vi "Launcher Template (Top Level VI).vi"() -> ()   [LabVIEW 2021]
uses:
  Typedefs/FGV Ref. Modules Function.ctl
  Typedefs/Enum_Module_Name.ctl
  Typedefs/Module References.ctl
  Typedefs/Message.ctl
  Modules/Configuration/Main Config.vi
  Modules/Core UI/SubVIs/Main Core UI.vi
  Modules/Module Template/SubVIs/Main.vi
  Modules/Module Template/Module Template.lvlib
  Modules/Configuration/Configuration.lvlib
  Architecture.lvlib
  Modules/Core UI/Core UI.lvlib
panel:
  out "error out":errorcluster
  in  "Loading Bar":u8(slide) caption="Loading Database..." max=100 step=1 scale=0.0..100.0
  # "APPLICATION LAUNCHER"
  # "Juan Pérez Rodríguez"
  # "https://CtrlVIStudios.com"
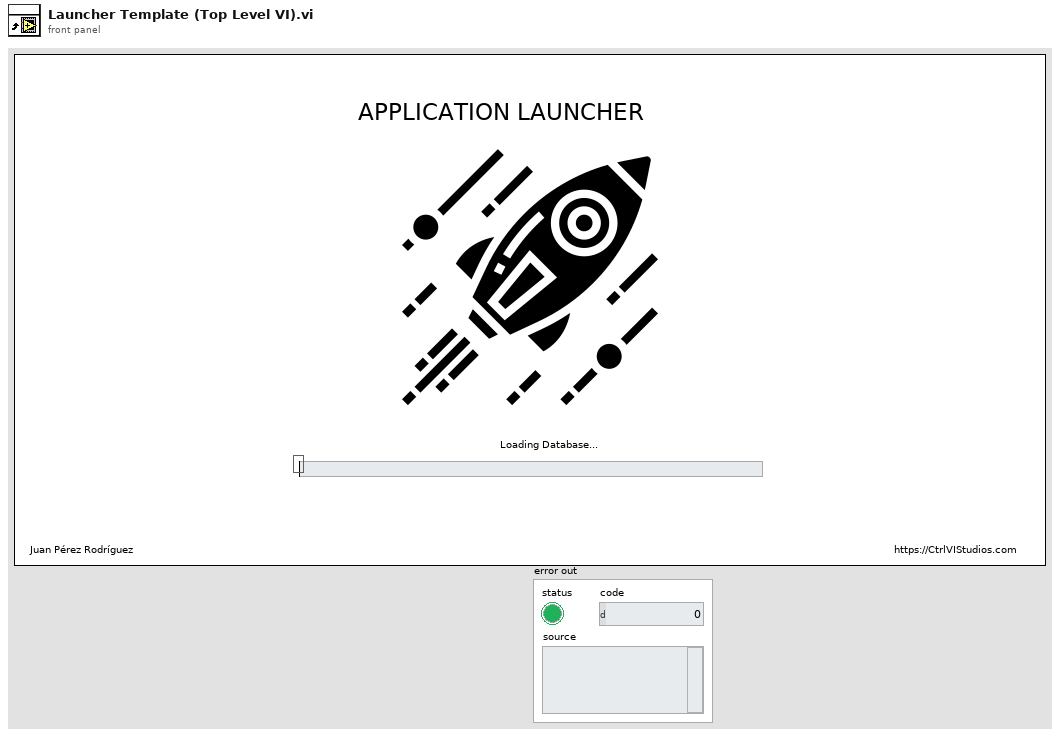
[diagram p1: front panel]
types:
  T1 = typedef "Configuration.lvlib/Enum_Module_Name.ctl" = enum16{"Configuration", "Error_Handler", "Log", "Database", "Controller", "UI Module"}
  T2 = cluster{"ModuleName":T1, "ShowFP":bool, "StatesTracking Enabled":bool}[]
  T3 = typedef "Architecture.lvlib/FGV Ref. Modules Function.ctl" = enum16{"Init ", "Add Module", "Get Module", "Get All", "Add Asynchronous Run Ref", "Dispose"}
  T4 = typedef "Architecture.lvlib/Module References.ctl" = cluster{"ModuleName":T1, "Queue":refnum<queue>, "user event":refnum<user-event>, "VI Refnum":refnum<vi>, "ShowFP":bool, "StatesTracking Enabled":bool}
  T5 = enum32{"invalid app kind", "Development System", "Run Time System", "Student Edition", "Embedded LabVIEW", "Evaluation", "Custom"}
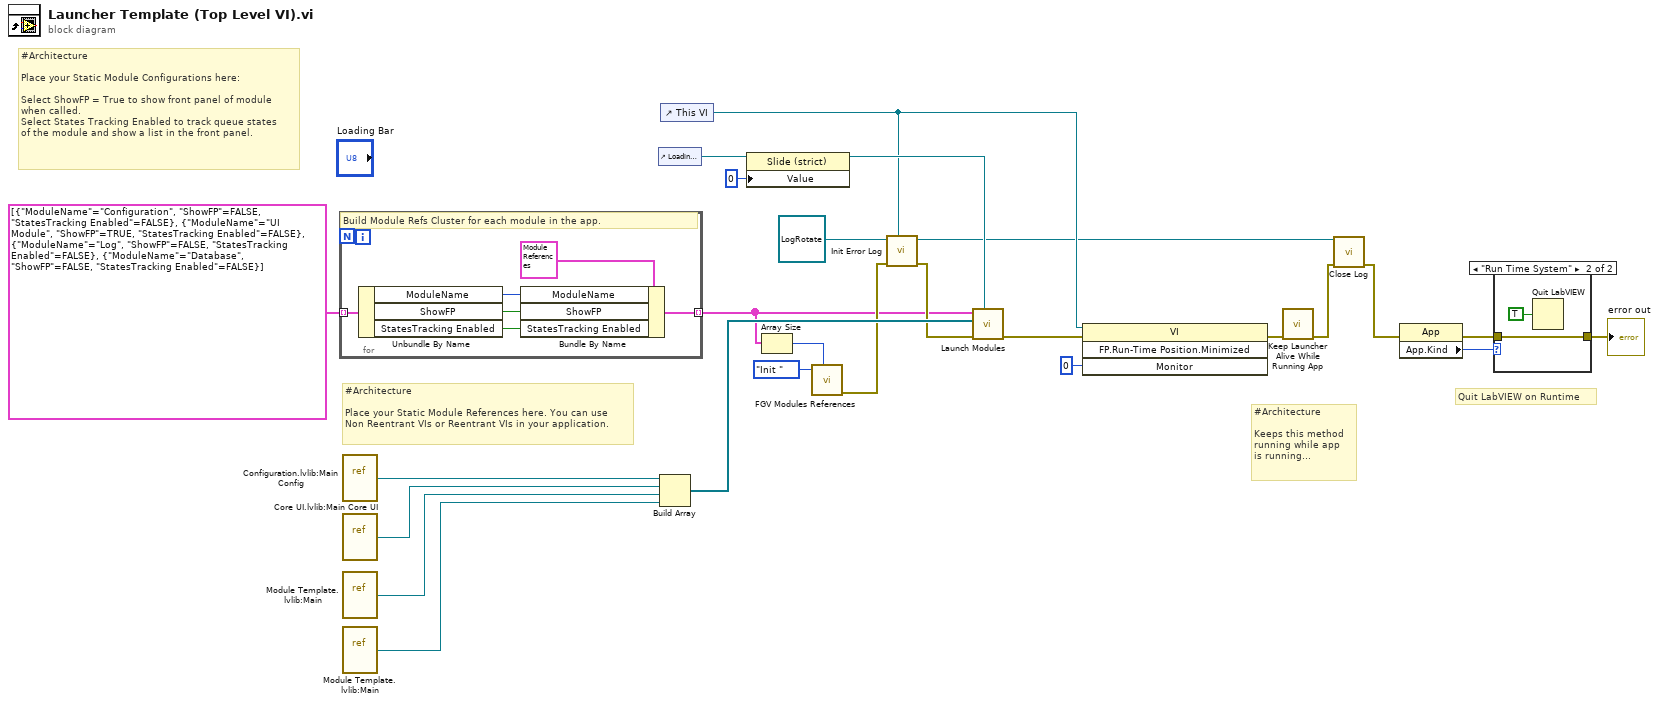
[diagram p0: block diagram]
diagram:
  # "#Architecture\n\nKeeps this method \nrunning while app \nis running..."
  # "Quit LabVIEW on Runtime"
  # "#Architecture\n\nPlace your Static Module References here. You can use\nNon Reentrant VIs or Reentrant VIs in your application."
  # "#Architecture\n\nPlace your Static Module Configurations here:\n\nSelect ShowFP = True to show front panel of module\nwhen called. \nSelect States Tracking Enabled to track queue states\nof the module and show a list in the front panel."
  n1 = for {
    tunnel: T2 [{"ModuleName"=enum."Configuration", "ShowFP"=FALSE, "StatesTracking Enabled"=FALSE}, {"ModuleName"=enum."UI Module", "ShowFP"=TRUE, "StatesTracking Enabled"=FALSE}, {"ModuleName"=enum."Log", "ShowFP"=FALSE, "StatesTracking Enabled"=FALSE}, {"ModuleName"=enum."Database", "ShowFP"=FALSE, "StatesTracking Enabled"=FALSE}] -> [w30] mode=indexing
    tunnel: [w26] -> w2 mode=indexing
    # "Build Module Refs Cluster for each module in the app."
    n2 = Unbundle By Name(w30) -> ("ModuleName"=w29:T1, "ShowFP"=w28:bool, "StatesTracking Enabled"=w27:bool)
    n3 = Bundle By Name(cluster=T4 {"ModuleName"=enum."Controller", "Queue"=refnum, "user event"=refnum, "VI Refnum"=refnum, "ShowFP"=FALSE, "StatesTracking Enabled"=FALSE} ("Module_Refs"), "ModuleName"=w29, "ShowFP"=w28, "StatesTracking Enabled"=w27) -> (w26:T4)
  }
  n4 = vi-ref "Configuration.lvlib:Main Config.vi"() -> (w16:refnum<vi>)
  n5 = vi-ref "Core UI.lvlib:Main Core UI.vi"() -> (w15:refnum<vi>)
  n6 = vi-ref "Module Template.lvlib:Main.vi"() -> (w14:refnum<vi>)
  n7 = vi-ref "Module Template.lvlib:Main.vi"() -> (w13:refnum<vi>)
  n8 = control-ref of="Loading Bar"() -> (w24:refnum<vi>)
  n9 = Build Array(w16, w15, w14, w13) -> (w19:refnum<vi>[])
  n10 = control-ref of="This VI"() -> (w6:refnum<vi>)
  n11 = property class="Slide (strict)"(reference=w24, "Value"=u8 0) -> (reference out=w22:refnum<vi>)  [unwired: 1 in, 1 out]
  n12 = Array Size(array=w2) -> (size(s)=w1:i32)
  n13 = call "FGV Modules References.vi"("size(s)"=w1, "FGV Ref. Function In"=FGV_Ref._Modules_Function."Init ") -> ("error out"=w9:errorcluster)  [unwired: 6 in, 3 out]
  n14 = call "Init Error Log.vi"("TopLevel"=w6, "error in (no error)"=w9, "LogRotate in"=refnum<class "LogRotate.lvclass"> refnum) -> ("error out"=w8:errorcluster, "LogRotate out"=w5:refnum<class "LogRotate.lvclass">)  [unwired: 7 in]
  n15 = call "Launch Modules.vi"("Loading Bar Ref In"=w22, "error in (no error)"=w8, "App Modules Refs"=w19, "Modules Info In"=w2) -> ("error out"=w20:errorcluster)  [unwired: 7 in]
  n16 = invoke class="VI" method="FP.Run-Time Position.Minimized"(reference=w6, error in=w20, "Monitor"=i16 0) -> (error out=w18:errorcluster)  [unwired: 1 in, 3 out]
  n17 = call "Keep Launcher Alive While Running App.vi"("error in (no error)"=w18) -> ("error out"=w4:errorcluster)  [unwired: 10 in]
  n18 = call "Close Log.vi"("error in (no error)"=w4, "LogRotate in"=w5) -> ("error out"=w3:errorcluster)  [unwired: 8 in, 1 out]
  n19 = property class="App"(error in=w3) -> (error out=w12:errorcluster, "App.Kind"=w10:T5)  [unwired: 1 in, 1 out]
  n20 = case shown="\"Run Time System\"" w10 {
    tunnel: w12 -> [w32 w34]
    tunnel: [w32 w34] -> w11
    frame Default {
    }
    frame "Run Time System" {
      n21 = Quit LabVIEW(quit? (T)=TRUE) -> ()
    }
  }
  "error out" <- w11
